vi "Out_S5F8.vi"(8 "error in (no error)":errorcluster, 10 "S5F8":T1[](array[typedef]), 11 "S5 Message Class in":refnum<class "S5 Message Class.lvclass">) -> (0 "error out":errorcluster, 3 "S5 Message Class out":refnum<class "S5 Message Class.lvclass">)   [LabVIEW 2020, in "SECS Communication.lvlib" / "S5 Message Class.lvclass"]
uses:
  S5 Message Class.lvclass
  D:/Dropbox/SECS/SECS_GEM v1.1.0/Com/SECS Communication/SECS-II Class/SECS-II Class.lvclass
  S5F8.ctl
  SECS-II Class/Data Message_List.vi
  SECS-II Class/Data Message_Binary.vi
  SECS-II Class/Data Message_U4.vi
  SECS-II Class/Data Message_ASCII.vi
  SECS-II Class/SECS-II Class.lvclass
  D:/Dropbox/SECS/SECS_GEM v1.1.0/Com/SECS Communication/S5 Message Class/S5 Message Class.lvclass
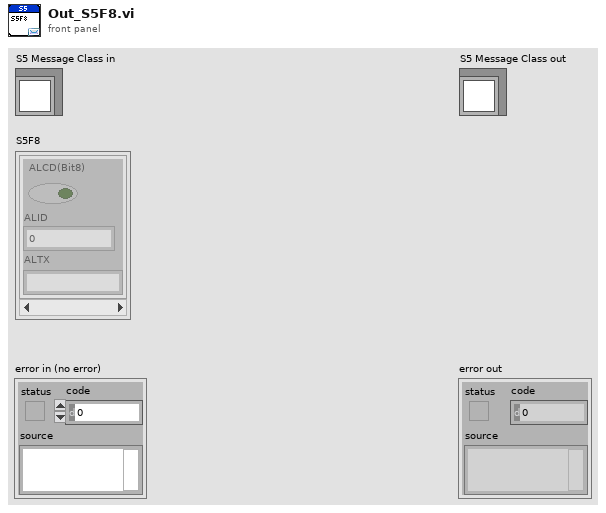
[diagram p1: front panel]
types:
  T1 = typedef "SECS Communication.lvlib/S5 Message Class.lvclass/S5F8.ctl" = cluster{"ALCD(Bit8)":bool, "ALID":u32, "ALTX":string}
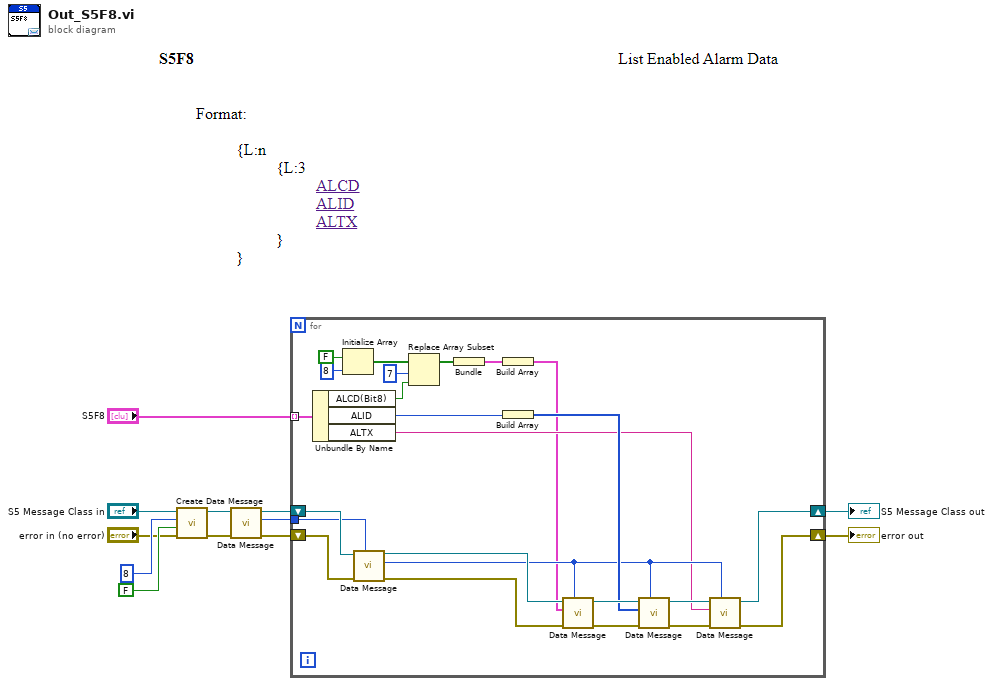
[diagram p0: block diagram]
diagram:
  n1 = call "Create Data Message.vi"("error in (no error)"="error in (no error)", "W-Bit"=FALSE, "Function"=u8 8, "SECS-II Class in"="S5 Message Class in") -> ("error out"=w10:errorcluster, "SECS-II Class out"=w9:refnum<class "S5 Message Class.lvclass">)  [unwired: 6 in]
  n2 = call-poly "Data Message.vi"("error in"=w10, "SECS-II Class in"=w9) -> ("error out"=w4:errorcluster, "Index"=w3:i32, "SECS-II Class out"=w5:refnum<class "S5 Message Class.lvclass">)  [unwired: 7 in]
  n3 = for {
    tunnel: "S5F8" -> [w32] mode=indexing
    tunnel: w3 -> [w34]
    shift-right: [w22] -> w2
    shift-left: w5 -> [w35]
    shift-right: [w21] -> w1
    shift-left: w4 -> [w36]
    n4 = Unbundle By Name(w32) -> ("ALCD(Bit8)"=w14:bool, "ALID"=w28:u32, "ALTX"=w23:string)
    n5 = Initialize Array(FALSE, 8 ("dimension size")) -> (w18:bool[])
    n6 = call-poly "Data Message.vi"("Parent Index"=w34, "error in"=w36, "SECS-II Class in"=w35) -> ("error out"=w31:errorcluster, "Index"=w24:i32, "SECS-II Class out"=w33:refnum<class "S5 Message Class.lvclass">)  [unwired: 6 in]
    n7 = Replace Array Subset(array=w18, new element=w14, index=7) -> (w16:bool[])
    n8 = Bundle(w16) -> (w15:cluster{bool[]})  [unwired: 1 in]
    n9 = Build Array(w15) -> (w13:cluster{bool[]}[])
    n10 = Build Array(w28) -> (w27:u32[])
    n11 = call-poly "Data Message.vi"("Parent Index"=w24, "error in"=w31, "Data Cluster"=w13, "SECS-II Class in"=w33) -> ("error out"=w29:errorcluster, "SECS-II Class out"=w30:refnum<class "S5 Message Class.lvclass">)  [unwired: 6 in]
    n12 = call-poly "Data Message.vi"("Parent Index"=w24, "error in"=w29, "Data"=w27, "SECS-II Class in"=w30) -> ("error out"=w25:errorcluster, "SECS-II Class out"=w26:refnum<class "S5 Message Class.lvclass">)  [unwired: 6 in]
    n13 = call-poly "Data Message.vi"("Parent Index"=w24, "error in"=w25, "Data"=w23, "SECS-II Class in"=w26) -> ("error out"=w21:errorcluster, "SECS-II Class out"=w22:refnum<class "S5 Message Class.lvclass">)  [unwired: 6 in]
  }
  "error out" <- w1
  "S5 Message Class out" <- w2
